vi "cnc-temperature.vi"(2 "speed in":i32(listbox), 3 "Temperature in":dbl(slide) scale=0.0..200.0) -> (1 "Temperature out":dbl(slide) scale=0.0..200.0)   [LabVIEW 2026]
uses:
  <vilib>/numeric/Random Number (Range) DBL.vi
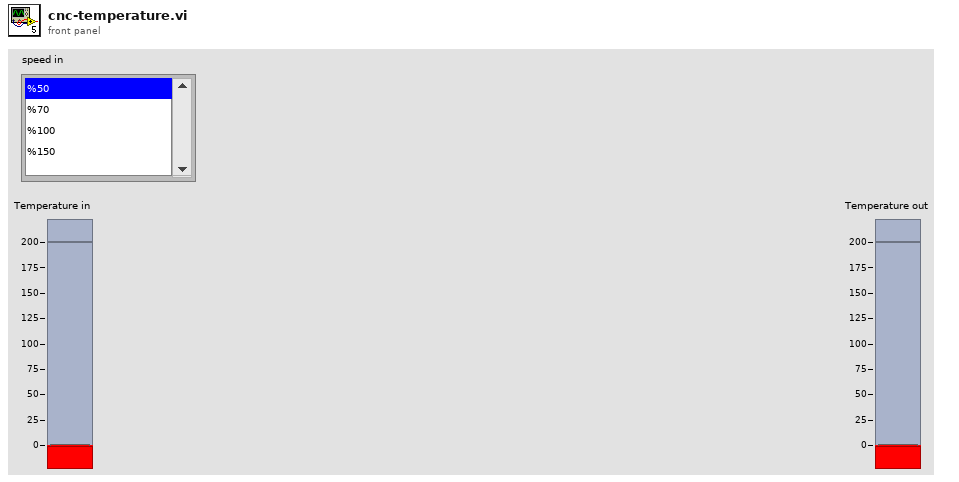
[diagram p1: front panel]
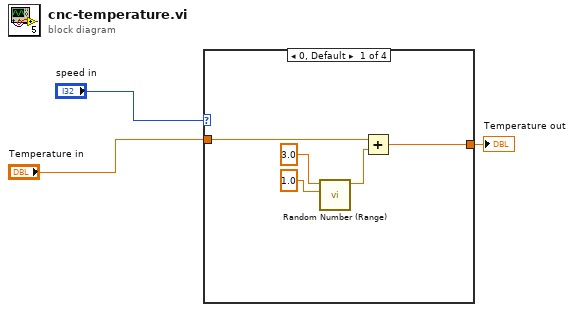
[diagram p0: block diagram]
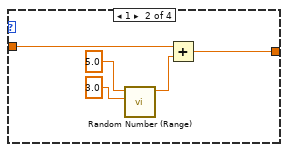
[diagram p2: hidden frame]
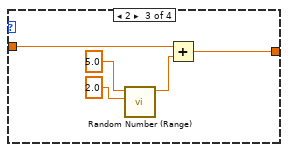
[diagram p3: hidden frame]
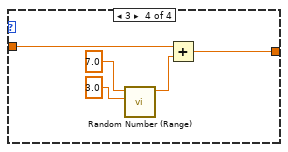
[diagram p4: hidden frame]
diagram:
  n1 = case shown="0, Default" "speed in" {
    tunnel: "Temperature in" -> [w5 w10 w15 w20]
    tunnel: [w4 w9 w14 w19] -> w1
    frame 0, Default {
      n2 = call-poly <vilib>:"Random Number (Range).vi"("lower bound (0)"=1.0, "upper bound (100)"=3.0) -> ("number"=w6:dbl)  [unwired: 9 in]
      n3 = Add(x=w5, y=w6) -> (x+y=w4:dbl)
    }
    frame 1 {
      n4 = call-poly <vilib>:"Random Number (Range).vi"("lower bound (0)"=3.0, "upper bound (100)"=5.0) -> ("number"=w13:dbl)  [unwired: 9 in]
      n5 = Add(x=w10, y=w13) -> (x+y=w9:dbl)
    }
    frame 2 {
      n6 = call-poly <vilib>:"Random Number (Range).vi"("lower bound (0)"=2.0, "upper bound (100)"=5.0) -> ("number"=w18:dbl)  [unwired: 9 in]
      n7 = Add(x=w15, y=w18) -> (x+y=w14:dbl)
    }
    frame 3 {
      n8 = call-poly <vilib>:"Random Number (Range).vi"("lower bound (0)"=3.0, "upper bound (100)"=7.0) -> ("number"=w23:dbl)  [unwired: 9 in]
      n9 = Add(x=w20, y=w23) -> (x+y=w19:dbl)
    }
  }
  "Temperature out" <- w1
